vi "Lista Servicios.vi"(11 "Servicio":string) -> (3 "Listado Servicios":string[](array[string]))   [LabVIEW 2020, in "Manejador Turnos.lvlib"]
uses:
  Manejador Turnos.lvlib
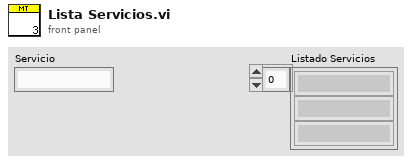
[diagram p1: front panel]
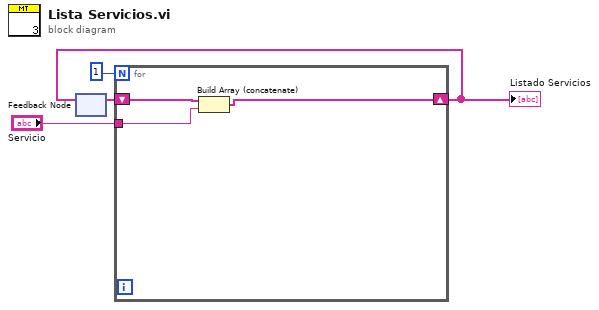
[diagram p0: block diagram]
diagram:
  n1 = feedback #1() -> (w3:string[])  [unwired: 1 in]
  n2 = for {
    N: 1 -> [_]
    shift-right: [w7] -> w1
    shift-left: w3 -> [w6]
    tunnel: "Servicio" -> [w5]
    n3 = Build Array (concatenate)(w6, w5) -> (w7:string[])
  }
  "Listado Servicios" <- w1
  n4 = feedback-in #1(w1) -> ()
